vi "Serial Port Read 2.vi"(8 "requested byte count":u32, 11 "port number":i32) -> (0 "error code":i32 format="%.0x", 1 "string read":string, 3 "port number out":i32)   [LabVIEW 2010]
doc: "Reads the number of characters specified by requested byte count from the serial port indicated in port number."
uses:
  <vilib>/Instr/serial.llb/serpConfig.vi
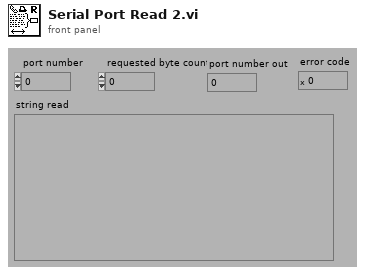
[diagram p1: front panel]
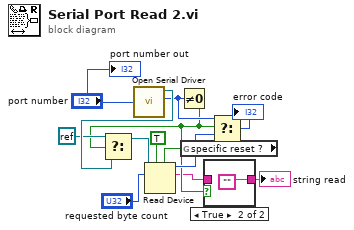
[diagram p0: block diagram]
diagram:
  n1 = call <vilib>:"Open Serial Driver.vi"("port number"="port number") -> ("input refnum"=w11:refnum<visa-resource-name>, "input error"=w7:i32)  [unwired: 2 out]
  n2 = Not Equal To 0?(x=w7) -> (x != 0?=w4:bool)
  n3 = Select(t=refnum<k0> refnum, s=w4, f=w11) -> (s? t:f=w9:refnum<visa-resource-name>)
  n4 = global read "serpConfig.vi" "specific reset ?"() -> (w3:bool)
  n5 = Read Device(4:w3, 6:TRUE, 9:"requested byte count", 10:w9) -> (2:w1:string, 3:w6:i16)  [unwired: 3 in, 1 out]
  n6 = case shown="True" w4 {
    tunnel: [w14 ""] -> w2
    tunnel: w1 -> [w14 _]
    frame False {
    }
    frame True {
    }
  }
  "string read" <- w2
  n7 = Select(t=w7, s=w4, f=w6) -> (s? t:f=→"error code":i32)
  "port number out" <- "port number"
